vi "TLPM Measure Power.vi"(8 "error in (no error)":errorcluster {"code" format="%.0x"}, 11 "instrument handle":refnum<visa-resource-name>) -> (0 "error out":errorcluster {"code" format="%.0x"}, 2 "Power":dbl, 3 "instrument handle out":refnum<visa-resource-name>)   [LabVIEW 2017]
doc: "This VI is used to obtain power readings from the instrument. \n\nRemark:\nThis VI starts a new measurement cycle and after finishing measurement the result is received. Subject to the actual Average Count this may take up to seconds. Refer to <Set/Get Average Count>."
uses:
  TLPM_64.dll
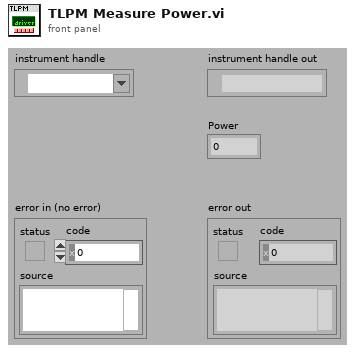
[diagram p1: front panel]
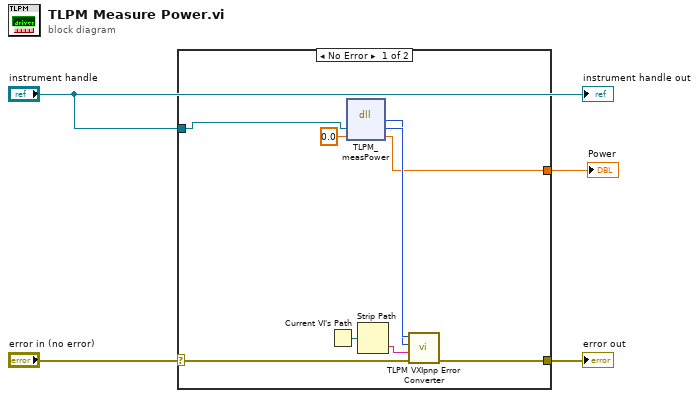
[diagram p0: block diagram]
diagram:
  n1 = case shown="No Error" "error in (no error)" {
    selector: "error in (no error)" -> [w8 w14]
    tunnel: [w7 w14] -> w4
    tunnel: "instrument handle" -> [w12 _]
    tunnel: [w5 _] -> w1
    frame No Error {
      n2 = Current VI's Path() -> (path=w13:path)
      n3 = dll-call lib="TLPM_64.dll" fn="TLPM_measPower"("Instrument Handle"=w12, "Power"=0.0) -> (w10:i32, "Instrument Handle"=w11:u32, "Power"=w5:dbl)  [unwired: 3 in, 2 out]
      n4 = Strip Path(path=w13) -> (name=w9:string)  [unwired: 1 out]
      n5 = call "TLPM VXIpnp Error Converter.vi"("error in (no error)"=w8, "Name Of VI (\"\")"=w9, "CVI Error Code (0)"=w10, "instrument handle"=w11) -> ("error out"=w7:errorcluster)  [unwired: 6 in, 1 out]
    }
    frame Error {
    }
  }
  "error out" <- w4
  "Power" <- w1
  "instrument handle out" <- "instrument handle"
